vi "Get Domain.vi"(8 "error in (no error)":errorcluster, 11 "Domain_Evolut_1D in":refnum<class "NI_Domain_Evolut_1D.lvclass">) -> (0 "error out":errorcluster, 2 "domain":variant, 3 "Domain_Evolut_1D out":refnum<class "NI_Domain_Evolut_1D.lvclass">)   [LabVIEW 2020, in "NI_PDE.lvlib" / "NI_Domain_Evolut_1D.lvclass"]
uses:
  <vilib>/gmath/pde.llb/DomainClass/Domain_Evolut_1D/NI_Domain_Evolut_1D.lvclass
  <vilib>/gmath/pde.llb/DomainClass/Domain_Evolut_1D/Domain Data.ctl
  <vilib>/gmath/pde.llb/DomainClass/Domain_Evolut_1D/NI_Domain_Evolut_1D.lvclass/NI_Domain_Evolut_1D.ctl
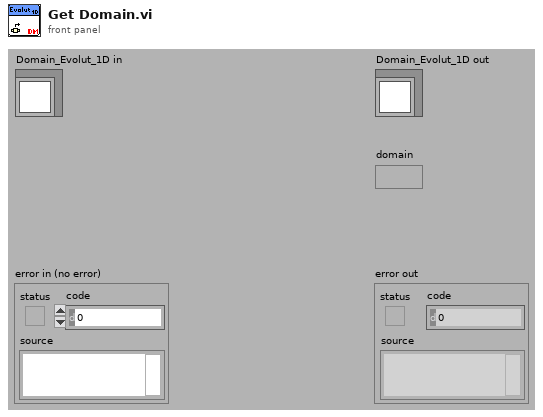
[diagram p1: front panel]
types:
  T1 = typedef "NI_PDE.lvlib/NI_Domain_Evolut_1D.lvclass/Domain Data.ctl" = cluster{"T":cluster{"initial t":dbl, "final t":dbl, "# of t-points":i32}, "X":cluster{"start x":dbl, "end x":dbl, "# of x-points":i32}}
  T2 = cluster{"initial t":dbl, "final t":dbl, "# of t-points":i32}
  T3 = cluster{"start x":dbl, "end x":dbl, "# of x-points":i32}
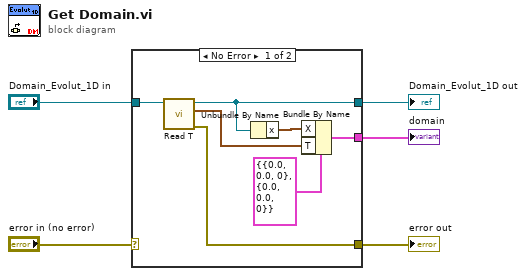
[diagram p0: block diagram]
diagram:
  n1 = case shown="No Error" "error in (no error)" {
    selector: "error in (no error)" -> [_ w14]
    tunnel: "Domain_Evolut_1D in" -> [w9 w13]
    tunnel: [w8 w13] -> w5
    tunnel: [w12 w14] -> w4
    tunnel: [w10 _] -> w1
    frame No Error {
      n2 = call-dynamic "Read T.vi"("Domain_Evolut.lvclass in"=w9) -> ("error out"=w12:errorcluster, "t"=w6:T2, "Domain_Evolut.lvclass out"=w8:refnum<class "NI_Domain_Evolut_1D.lvclass">)  [unwired: 1 in, 7 out]
      n3 = Unbundle By Name(w8) -> ("x"=w7:T3)
      n4 = Bundle By Name(cluster=T1 {"T"={"initial t"=0.0, "final t"=0.0, "# of t-points"=0}, "X"={"start x"=0.0, "end x"=0.0, "# of x-points"=0}} ("domain data"), "X"=w7, "T"=w6) -> (w10:T1)
    }
    frame Error {
    }
  }
  "Domain_Evolut_1D out" <- w5
  "error out" <- w4
  "domain" <- w1
